vi "Add Object Entry.vi"(8 "error in":errorcluster, 10 "Obj Entry":refnum<class "Object Entry.lvclass">, 11 "Obj Dict in":refnum<class "Object Dictionary.lvclass">) -> (0 "error out":errorcluster, 3 "Obj Dict out":refnum<class "Object Dictionary.lvclass">)   [LabVIEW 2020, in "CANopen.lvlib" / "Object Dictionary.lvclass"]
doc: "Adds an entry with the specified key and value into the Object Dictionary collection with the lowest available index."
uses:
  Object Dictionary.lvclass
  Object Entry/Object Entry.lvclass
  Object Dictionary.lvclass/Object Dictionary.ctl
  Ordered-Dictionary/Ordered Object Dictionary/Source/Ordered Object Dictionary.lvclass
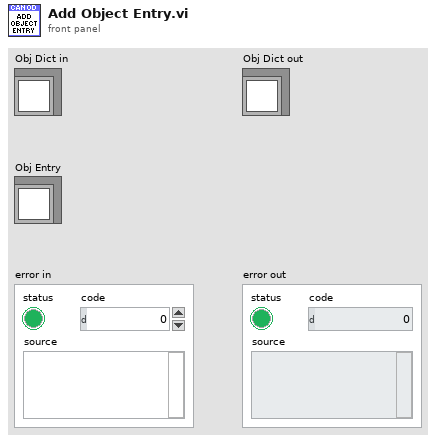
[diagram p1: front panel]
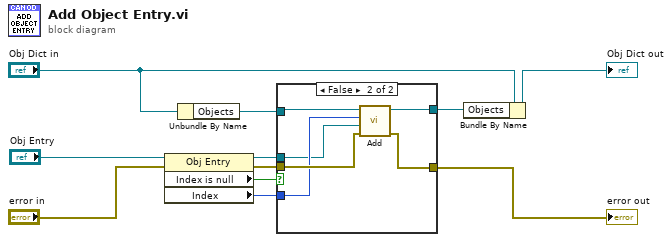
[diagram p0: block diagram]
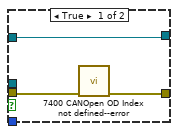
[diagram p2: hidden frame]
diagram:
  n1 = property class="Obj Entry"(reference="Obj Entry", error in="error in") -> (reference out=w2:refnum<class "Object Entry.lvclass">, error out=w4:errorcluster, "Index is null"=w5:bool, "Index"=w3:u16)
  n2 = Unbundle By Name("Obj Dict in") -> ("Objects"=w6:refnum<class "Ordered Object Dictionary.lvclass">)
  n3 = case shown="False" w5 {
    tunnel: w6 -> [w14 w20]
    tunnel: w4 -> [w13 w19]
    tunnel: w3 -> [_ w18]
    tunnel: w2 -> [_ w17]
    tunnel: [w12 w16] -> w8
    tunnel: [w14 w15] -> w1
    frame True {
      n4 = call "7400 CANOpen OD Index not defined--error.vi"("error in"=w13) -> ("error out"=w12:errorcluster)  [unwired: 9 in, 1 out]
    }
    frame False {
      n5 = call "Add.vi"("error in"=w19, "Value"=w17, "Key"=w18, "Ordered Object Dictionary in"=w20) -> ("error out"=w16:errorcluster, "Ordered Object Dictionary out"=w15:refnum<class "Ordered Object Dictionary.lvclass">)  [unwired: 6 in]
    }
  }
  "error out" <- w8
  n6 = Bundle By Name(cluster="Obj Dict in", "Objects"=w1) -> (→"Obj Dict out":refnum<class "Object Dictionary.lvclass">)
